vi "drawImage.vi"(0 "reference":refnum<class "Graphics.lvclass">, 1 "Point":T2 {"y" format="%.2f"; "x" format="%.2f"}, 2 "lImagePath":path, 3 "MaskColor":u32=33554432 format="%.0x", 4 "Image":T1, 5 "error in (no error)":errorcluster, 6 "PointInCenter(UpperRightCorner=F)":bool) -> (14 "reference out":refnum<class "Graphics.lvclass">, 19 "error out":errorcluster)   [LabVIEW 2014, in "Graphics.lvclass"]
uses:
  <resource>/Framework/Providers/Open_GDS/UML/Graphics_class/Graphics.lvclass
  <resource>/Framework/Providers/Open_GDS/UML/General/Point/Point Point2D.ctl
  <vilib>/picture/picture.llb/imagedata.ctl
  <resource>/Framework/Providers/Open_GDS/UML/General/Rectangle/Rectangle Rectangle2D.ctl
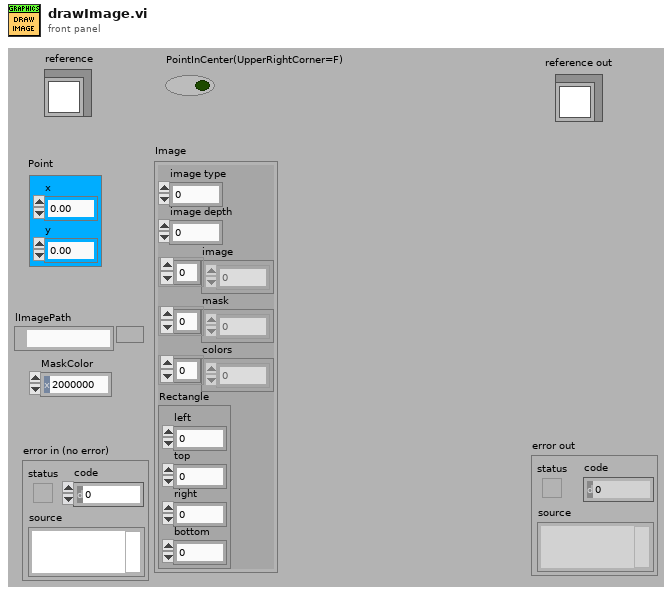
[diagram p1: front panel]
types:
  T1 = typedef "imagedata.ctl" = cluster{"image type":i32, "image depth":i32, "image":u8[], "mask":u8[], "colors":u32[], "Rectangle":cluster{"left":i16, "top":i16, "right":i16, "bottom":i16}}
  T2 = typedef "Point Point2D.ctl" = cluster{"x":dbl, "y":dbl}
  T3 = typedef "Rectangle Rectangle2D.ctl" = cluster{"x":dbl, "y":dbl, "width":dbl, "height":dbl}
  T4 = cluster{"left":i16, "top":i16, "right":i16, "bottom":i16}
  T5 = typedef "Graphics.lvclass/ObjectAttributes.ctl" = cluster{"drawColor":u32, "backgroundColor":u32, "font":T6, "fontType":T7, "picture":picture, "stroke":T8, "scaleX":dbl, "scaleY":dbl, "screenRef":refnum<vi>, "offsetX":dbl, "offsetY":dbl}
  T6 = typedef "Graphics.lvclass/FontType.ctl" = cluster{"Font Name:":string, "Size":i16, "Strikeout?":bool, "Italic?":bool, "Underline?":bool, "Outline?":bool, "Shadow?":bool, "Bold?":bool}
  T7 = typedef "Graphics.lvclass/LvFontType.ctl" = enum16{"User-specified Font", "Application Font", "System Font", "Dialog Font"}
  T8 = typedef "Graphics.lvclass/StrokeType.ctl" = enum16{"USE_DEFAULT", "SOLID", "DOTTED"}
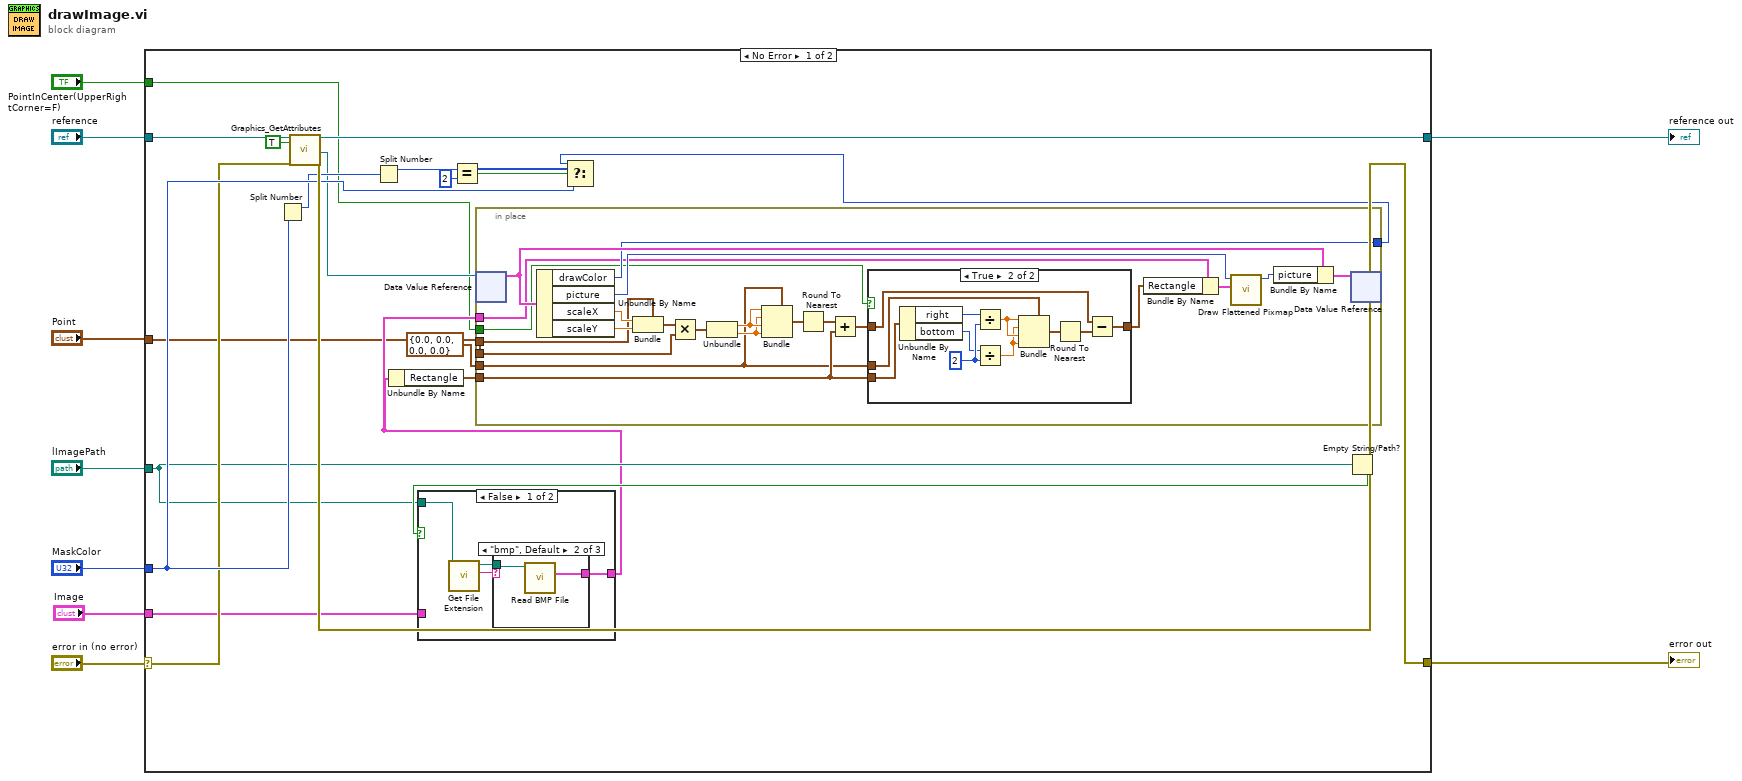
[diagram p0: block diagram]
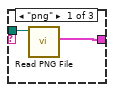
[diagram p3: hidden frame]
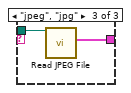
[diagram p4: hidden frame]
diagram:
  n1 = case shown="No Error" "error in (no error)" {
    selector: "error in (no error)" -> [w25 w75]
    tunnel: "reference" -> [w29 w76]
    tunnel: [w28 w75] -> w8
    tunnel: [w27 w76] -> w7
    tunnel: "Point" -> [w13 _]
    tunnel: "lImagePath" -> [w18 _]
    tunnel: "MaskColor" -> [w26 _]
    tunnel: "Image" -> [w19 _]
    tunnel: "PointInCenter(UpperRightCorner=F)" -> [w12 _]
    frame No Error {
      n2 = Split Number(x=w26) -> (hi(x)=w24:u16)  [unwired: 1 out]
      n3 = call <resource>:"Graphics_GetAttributes.vi"("reference in"=w29, "OnlyGetDvrReference(False)"=TRUE, "error in (no error)"=w25) -> ("reference out"=w27:refnum<class "Graphics.lvclass">, "DataRef"=w16:refnum<data-value>, "error out"=w28:errorcluster)  [unwired: 13 in, 1 out]
      n4 = Split Number(x=w24) -> (hi(x)=w23:u8)  [unwired: 1 out]
      n5 = Equal?(x=w23, y=u8 2) -> (x = y?=w21:bool)
      n6 = Empty String/Path?(string/path=w18) -> (empty?=w20:bool)
      n7 = case shown="False" w20 {
        tunnel: [w65 w74] -> w14
        tunnel: w18 -> [w64 _]
        tunnel: w19 -> [_ w74]
        frame False {
          n8 = call <vilib>:"Get File Extension.vi"("file"=w64) -> ("lowercase file extension"=w67:string, "dup file"=w66:path)  [unwired: 1 in, 8 out]
          n9 = case shown="\"bmp\", Default" w67 {
            tunnel: w66 -> [w69 w71 w73]
            tunnel: [w68 w70 w72] -> w65
            frame "png" {
              n10 = call <vilib>:"Read PNG File.vi"("path to PNG file"=w69) -> ("image data"=w68:T1)  [unwired: 1 in, 9 out]
            }
            frame "bmp", Default {
              n11 = call <vilib>:"Read BMP File.vi"("path to BMP file"=w71) -> ("image data"=w70:T1)  [unwired: 1 in, 9 out]
            }
            frame "jpeg", "jpg" {
              n12 = call <vilib>:"Read JPEG File.vi"("path to JPEG file"=w73) -> ("image data"=w72:T1)  [unwired: 1 in, 9 out]
            }
          }
        }
        frame True {
        }
      }
      n13 = Unbundle By Name(w14) -> ("Rectangle"=w11:T4)
      n14 = in-place {
        in-place-border: [w48] -> w15
        in-place-border: w13 -> [w43]
        in-place-border: w14 -> [w41]
        in-place-border: w13 -> [w39]
        in-place-border: w12 -> [w37]
        in-place-border: w11 -> [w33]
        in-place-border: T3 {"x"=0.0, "y"=0.0, "width"=0.0, "height"=0.0} ("x") -> [w31]
        n15 = in-place-dvr #1(w16) -> (w51:T5)  [unwired: 1 out]
        n16 = Unbundle By Name(w51) -> ("drawColor"=w48:u32, "picture"=w47:picture, "scaleX"=w46:dbl, "scaleY"=w45:dbl)
        n17 = Bundle(cluster=w43, "x"=w46, "y"=w45) -> (w42:T2)
        n18 = Multiply(x=w42, y=w39) -> (x*y=w38:T2)
        n19 = Unbundle(w38) -> ("x"=w35:dbl, "y"=w34:dbl)
        n20 = Bundle(cluster=w31, "x"=w35, "y"=w34, "width"=w35, "height"=w34) -> (w30:T3)
        n21 = Round To Nearest(number=w30) -> (nearest integer value=w32:T3)
        n22 = Add(x=w32, y=w33) -> (x+y=w36:T3)
        n23 = case shown="True" w37 {
          tunnel: w33 -> [_ w63]
          tunnel: w36 -> [w52 w61]
          tunnel: [w52 w54] -> w40
          tunnel: w31 -> [_ w60]
          frame False {
          }
          frame True {
            w62 = i16 2 ("y")
            n24 = Unbundle By Name(w63) -> ("right"=w58:i16, "bottom"=w57:i16)
            n25 = Divide(x=w58, y=w62) -> (x/y=w56:dbl)
            n26 = Divide(x=w57, y=w62) -> (x/y=w55:dbl)
            n27 = Bundle(cluster=w60, "x"=w56, "y"=w55, "width"=w56, "height"=w55) -> (w59:T3)
            n28 = Round To Nearest(number=w59) -> (nearest integer value=w53:T3)
            n29 = Subtract(x=w61, y=w53) -> (x-y=w54:T3)
          }
        }
        n30 = Bundle By Name(cluster=w41, "Rectangle"=w40) -> (w44:T1)
        n31 = call <vilib>:"Draw Flattened Pixmap.vi"("image data"=w44, "picture"=w47) -> ("new picture"=w50:picture)  [unwired: 2 in, 5 out]
        n32 = Bundle By Name(cluster=w51, "picture"=w50) -> (w49:T5)
        n33 = in-place-dvr #1(w49) -> ()  [unwired: 2 out]
      }
      n34 = Select(t=w15, s=w21, f=w26) -> ()  [unwired: 1 out]
    }
    frame Error {
    }
  }
  "reference out" <- w7
  "error out" <- w8
